vi "2048 Main.vi"() -> ()   [LabVIEW 2016]
uses:
  Board/Board.lvclass
  <vilib>/LIEF/Image Editor Handler/Send RemoveShapeByRef Event.vi
  <vilib>/LIEF/Image Editor Handler/Image Editor Handler.lvclass
  <vilib>/LIEF/Forms/Grid/Grid.lvclass
panel:
  in  "2D Picture":picture
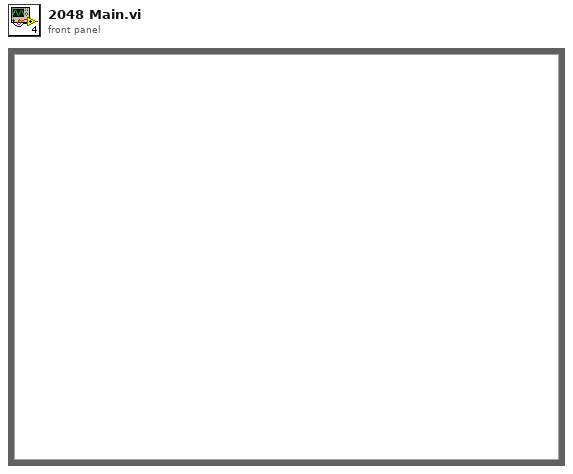
[diagram p1: front panel]
types:
  T1 = enum32{"invalid app kind", "Development System", "Run Time System", "Student Edition", "Embedded LabVIEW", "Evaluation", "Custom"}
  T2 = typedef "LVBoundsTypeDef.ctl" = cluster{"Width":u32, "Height":u32}
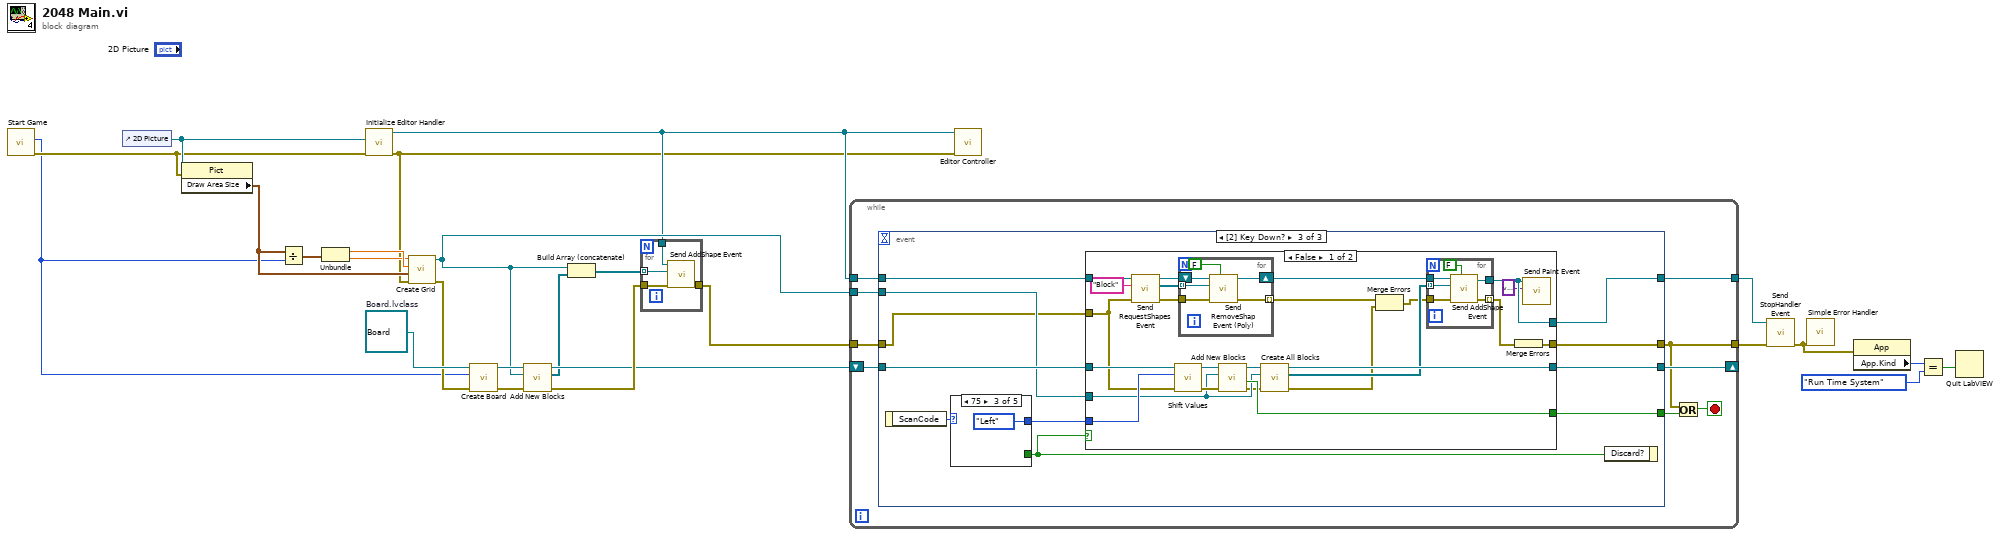
[diagram p0: block diagram]
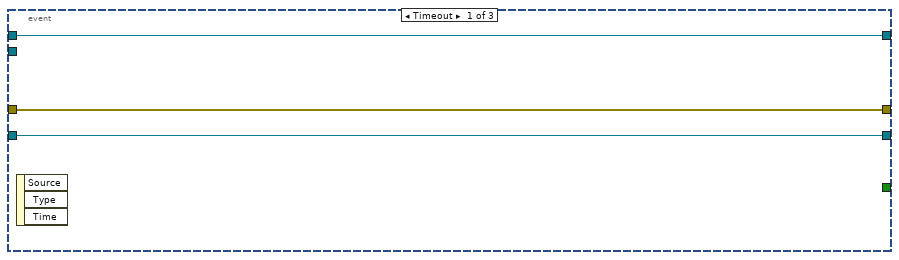
[diagram p2: hidden frame]
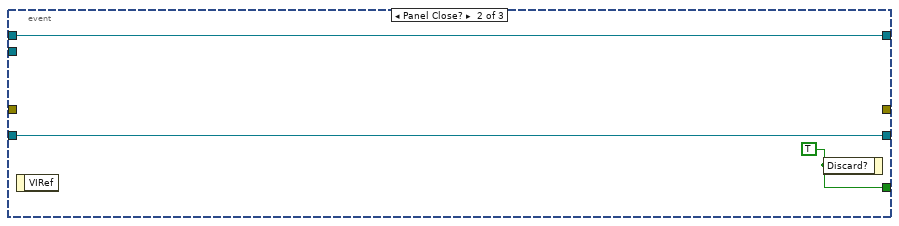
[diagram p3: hidden frame]
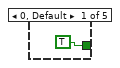
[diagram p5: hidden frame]
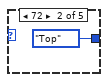
[diagram p6: hidden frame]
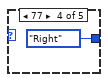
[diagram p7: hidden frame]
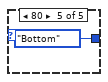
[diagram p8: hidden frame]
diagram:
  w20 = refnum<class "Board.lvclass"> refnum  # Board.lvclass
  n1 = call "Start Game.vi"() -> ("error out"=w6:errorcluster, "Board Size out"=w5:i16)  [unwired: 10 in]
  n2 = control-ref of="2D Picture"() -> (w25:refnum<vi>)
  n3 = property class="Pict"(reference=w25, error in=w6) -> ("Draw Area Size"=w19:T2)  [unwired: 2 out]
  n4 = Divide(x=w19, y=w5) -> (x/y=w18:cluster{"Width":dbl, "Height":dbl})
  n5 = Unbundle(w18) -> ("Width"=w24:dbl, "Height"=w23:dbl)
  n6 = call <vilib>:"Initialize Editor Handler.vi"("error in (no error)"=w6, "PictureRef"=w25) -> ("error out"=w10:errorcluster, "Editor Handler out"=w12:refnum<class "Image Editor Handler.lvclass">)  [unwired: 8 in]
  n7 = call <vilib>:"Create Grid.vi"("error in (no error)"=w10, "Draw Area"=w19, "Horizontal Step"=w24, "Vertical Step"=w23) -> ("error out"=w17:errorcluster, "Grid Reference"=w13:refnum<data-value>)  [unwired: 6 in]
  n8 = call "Create Board.vi"("error in (no error)"=w17, "Board Size"=w5, "Board in"=w20) -> ("error out"=w16:errorcluster, "Board out"=w21:refnum<class "Board.lvclass">)  [unwired: 7 in]
  n9 = call "Add New Blocks.vi"("error in (no error)"=w16, "Grid"=w13, "Board in"=w21) -> ("error out"=w15:errorcluster, "New Shapes"=w11:refnum<data-value>[], "Board in 2"=w14:refnum<class "Board.lvclass">)  [unwired: 5 in, 1 out]
  n10 = Build Array (concatenate)(w13, w11) -> (w22:refnum<data-value>[])
  n11 = for {
    tunnel: w15 -> [w29]
    tunnel: w12 -> [w28]
    tunnel: w22 -> [w27] mode=indexing
    tunnel: [w26] -> w7
    n12 = call <vilib>:"Send AddShape Event.vi"("error in (no error)"=w29, "New Shape Reference"=w27, "Editor Handler in"=w28) -> ("error out"=w26:errorcluster)  [unwired: 7 in, 1 out]
  }
  n13 = while {
    tunnel: w12 -> [w37]
    shift-right: [w35] -> _
    shift-left: w14 -> [w36]
    tunnel: w13 -> [w34]
    tunnel: [w31] -> w9
    tunnel: [w33] -> w8
    tunnel: w7 -> [w30]
    stop <- w32 stop-if-true
    n14 = event shown="[2] Key Down?" {
      selector: _ -> [_ _ _]
      dyn-events: _ -> [_ _ _]
      timeout: _ -> [_ _ _]
      tunnel: [_ w44 w52] -> w38
      tunnel: w37 -> [w40 w42 w48]
      tunnel: w36 -> [w41 w43 w55]
      tunnel: [w41 w43 w53] -> w35
      tunnel: w34 -> [_ _ w54]
      tunnel: [w39 _ w47] -> w31
      tunnel: [w40 w42 w46] -> w33
      tunnel: w30 -> [w39 _ w45]
      event Timeout {
        n15 = event-data() -> ()  [unwired: 1 in, 3 out]
      }
      event Panel Close? {
        w44 = TRUE ("Discard?")
        n16 = event-data() -> ()  [unwired: 1 in, 1 out]
        n17 = event-data("Discard?"=w44) -> ()  [unwired: 1 in, 1 out]
      }
      event Key Down? {
        n18 = event-data() -> ("ScanCode"=w51:i16)  [unwired: 1 in]
        n19 = case shown="75" w51 {
          tunnel: [_ enum16{"Left", "Right", "Top", "Bottom"}."Top" ("Direction") enum16{"Left", "Right", "Top", "Bottom"}."Left" ("Direction") enum16{"Left", "Right", "Top", "Bottom"}."Right" ("Direction") enum16{"Left", "Right", "Top", "Bottom"}."Bottom" ("Direction")] -> w50
          tunnel: [TRUE _ _ _ _] -> w49
          frame 0, Default {
          }
          frame 72 {
          }
          frame 75 {
          }
          frame 77 {
          }
          frame 80 {
          }
        }
        n20 = case shown="False" w49 {
          tunnel: w55 -> [w79 w94]
          tunnel: w54 -> [w71 _]
          tunnel: [w72 w94] -> w53
          tunnel: [w76 _] -> w52
          tunnel: w50 -> [w75 _]
          tunnel: w48 -> [w74 w93]
          tunnel: [w65 w92] -> w47
          tunnel: [w57 w93] -> w46
          tunnel: w45 -> [w64 w92]
          frame False {
            n21 = call <vilib>:"Send RequestShapes Event.vi"("error in (no error)"=w64, "Shape Class Filter"="Block", "Editor Handler in"=w74) -> ("error out"=w61:errorcluster, "Shapes"=w62:refnum<data-value>[], "Editor Handler out"=w63:refnum<class "Image Editor Handler.lvclass">)  [unwired: 6 in]
            n22 = call "Shift Values.vi"("error in (no error)"=w64, "Direction"=w75, "Board in"=w79) -> ("error out"=w77:errorcluster, "Board out"=w78:refnum<class "Board.lvclass">)  [unwired: 7 in]
            n23 = for {
              tunnel: w62 -> [w84] mode=indexing
              tunnel: w61 -> [w83]
              shift-right: [w82] -> w60
              shift-left: w63 -> [w85]
              tunnel: [w81] -> w59 mode=indexing
              n24 = call-poly <vilib>:"Send RemoveShap Event (Poly).vi"("Auto-Refresh (T)"=FALSE, "error in (no error)"=w83, "Shape"=w84, "Editor Handler in"=w85) -> ("error out"=w81:errorcluster, "Editor Handler out"=w82:refnum<class "Image Editor Handler.lvclass">)  [unwired: 6 in]
            }
            n25 = call "Add New Blocks.vi"("error in (no error)"=w77, "Grid"=w71, "Board in"=w78) -> ("error out"=w69:errorcluster, "No Busy"=w76:bool, "Board in 2"=w73:refnum<class "Board.lvclass">)  [unwired: 5 in, 1 out]
            n26 = call "Create All Blocks.vi"("error in (no error)"=w69, "Grid"=w71, "Board in"=w73) -> ("error out"=w68:errorcluster, "New Blocks"=w70:refnum<data-value>[], "Board out"=w72:refnum<class "Board.lvclass">)  [unwired: 6 in]
            n27 = Merge Errors(w59, w68) -> (w67:errorcluster)
            n28 = for {
              tunnel: w67 -> [w91]
              tunnel: w60 -> [w90]
              tunnel: w70 -> [w89] mode=indexing
              tunnel: [w88] -> w66 mode=indexing
              tunnel: [w87] -> w57
              n29 = call <vilib>:"Send AddShape Event.vi"("Auto-Refresh (T)"=FALSE, "error in (no error)"=w91, "New Shape Reference"=w89, "Editor Handler in"=w90) -> ("error out"=w88:errorcluster, "Editor Handler out"=w87:refnum<class "Image Editor Handler.lvclass">)  [unwired: 6 in]
            }
            n30 = Merge Errors(w66) -> (w65:errorcluster)
            n31 = call <vilib>:"Send Paint Event.vi"("event data"=variant, "Editor Handler in"=w57) -> ()  [unwired: 8 in, 2 out]
          }
          frame True {
          }
        }
        n32 = event-data("Discard?"=w49) -> ()  [unwired: 1 in, 1 out]
      }
    }
    n33 = Or(x=w31, y=w38) -> (x .or. y?=w32:bool)
  }
  n34 = call <vilib>:"Editor Controller.vi"("error in (no error)"=w10, "Editor Handler in"=w12) -> ()  [unwired: 8 in, 2 out]
  n35 = call <vilib>:"Send StopHandler Event.vi"("error in (no error)"=w9, "Editor Handler in"=w8) -> ("error out"=w4:errorcluster)  [unwired: 8 in, 1 out]
  n36 = call <vilib>:"Simple Error Handler.vi"("error in (no error)"=w4) -> ()  [unwired: 4 in, 5 out]
  n37 = property class="App"(error in=w4) -> ("App.Kind"=w3:T1)  [unwired: 1 in, 2 out]
  n38 = Equal?(x=w3, y=T1."Run Time System") -> (x = y?=w1:bool)
  n39 = Quit LabVIEW(quit? (T)=w1) -> ()
